vi "Name to Symbol.vi"(11 "item name":string) -> (3 "item symbol":T1)   [LabVIEW 2020, in "Ballard MIL-STD-1553 System Explorer.lvlib" / "Implementation.lvlib" / "Refresh.lvlib"]
uses:
  Refresh.lvlib
  Symbols.ctl
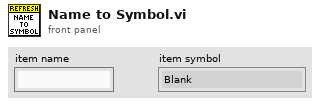
[diagram p1: front panel]
types:
  T1 = typedef "Ballard MIL-STD-1553 System Explorer.lvlib/Implementation.lvlib/Refresh.lvlib/Symbols.ctl" = enum16{"Blank", "MIL-STD-1553", "Port", "Remote Terminal", "Subaddress", "Bus Controller", "Acyclic Frame", "Mode Code", "Message", "Parameter", "Item"}
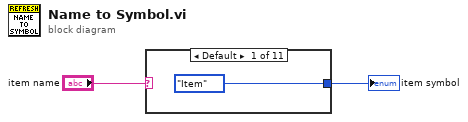
[diagram p0: block diagram]
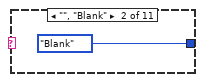
[diagram p2: hidden frame]
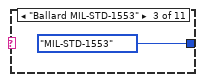
[diagram p3: hidden frame]
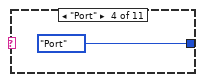
[diagram p4: hidden frame]
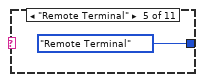
[diagram p5: hidden frame]
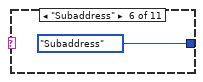
[diagram p6: hidden frame]
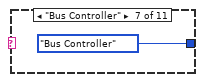
[diagram p7: hidden frame]
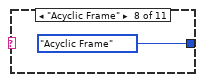
[diagram p8: hidden frame]
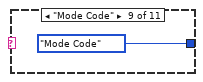
[diagram p9: hidden frame]
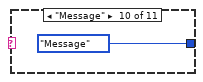
[diagram p10: hidden frame]
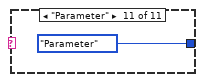
[diagram p11: hidden frame]
diagram:
  n1 = case shown="Default" "item name" {
    tunnel: [Symbols."Item" ("item symbol") Symbols."Blank" ("item symbol") Symbols."MIL-STD-1553" ("item symbol") Symbols."Port" ("item symbol") Symbols."Remote Terminal" ("item symbol") Symbols."Subaddress" ("item symbol") Symbols."Bus Controller" ("item symbol") Symbols."Acyclic Frame" ("item symbol") Symbols."Mode Code" ("item symbol") Symbols."Message" ("item symbol") Symbols."Parameter" ("item symbol")] -> w2
    frame Default {
    }
    frame "", "Blank" {
    }
    frame "Ballard MIL-STD-1553" {
    }
    frame "Port" {
    }
    frame "Remote Terminal" {
    }
    frame "Subaddress" {
    }
    frame "Bus Controller" {
    }
    frame "Acyclic Frame" {
    }
    frame "Mode Code" {
    }
    frame "Message" {
    }
    frame "Parameter" {
    }
  }
  "item symbol" <- w2
